vi "Construct Advanced Text Log Sink.vi"(7 "LogLevel":T3, 8 "StringFormat":refnum<class "IStringFormat.lvclass">, 9 "Log Filter":refnum<class "ILogFilter.lvclass">, 10 "Error Action":T1=enum."Ignore Error and Close Sink", 11 "Text File Configuration":T2={"Folder"=path "", "Name"="Event Log", "Extension"="txt", "Max Size (MB)"=1, "Timestamp Filename"=TRUE}) -> (3 "Text File Sink out":refnum<class "Text File Sink.lvclass">)   [LabVIEW 2018, in "MVA Framework.lvlib" / "Text File Sink.lvclass"]
doc: "Construct a text file sink. Text file configuration parameters are defined below.\n-Folder - the folder path where log files will be generated. If an empty path is supplied, a default folder path at public application data will be used.\n-Name - Name to give the log file. If no name is provided, a default file name cooresponding to the application directory name will be used.\n-Extension - file extension to be used for the log file. Note a period is not required here."
uses:
  Text File Sink.lvclass
  Composed Log/Log Sink/Log Sink.lvclass
  <vilib>/Utility/sysdir.llb/System Directory Type.ctl
  String Log Sink/String Log Sink.lvclass
  Composed Log/Types/Log Level.ctl
  Composed Log/Composed Log.lvlib
  Configuration.ctl
  Composed Log/Log Sink/Sink Error Actions ENUM.ctl
  Composed Log/ILogFilter/ILogFilter.lvclass
  IStringFormat/IStringFormat.lvclass
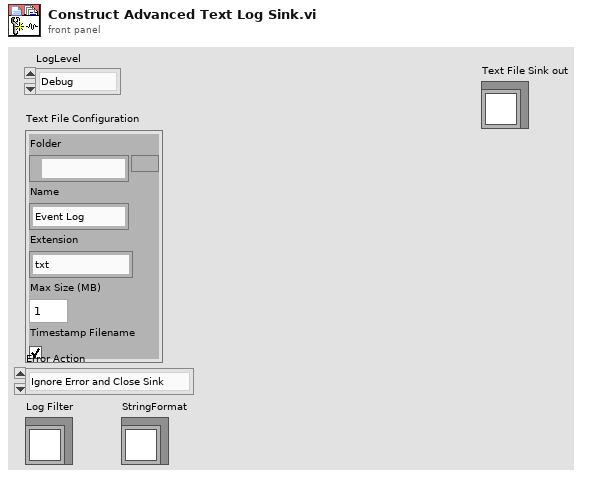
[diagram p1: front panel]
types:
  T1 = typedef "MVA Framework.lvlib/Composed Log.lvlib/Log Sink.lvclass/Sink Error Actions ENUM.ctl" = enum16{"Ignore Error and Continue", "Ignore Error and Close Sink", "Report Error and Close Sink"}
  T2 = typedef "MVA Framework.lvlib/Text File Sink.lvclass/Configuration.ctl" = cluster{"Folder":path, "Name":string, "Extension":string, "Max Size (MB)":i64, "Timestamp Filename":bool}
  T3 = typedef "MVA Framework.lvlib/Composed Log.lvlib/Log Level.ctl" = enum16{"Debug", "Info", "Warning", "Error", "Critical"}
  T4 = typedef "System Directory Type.ctl" = i32
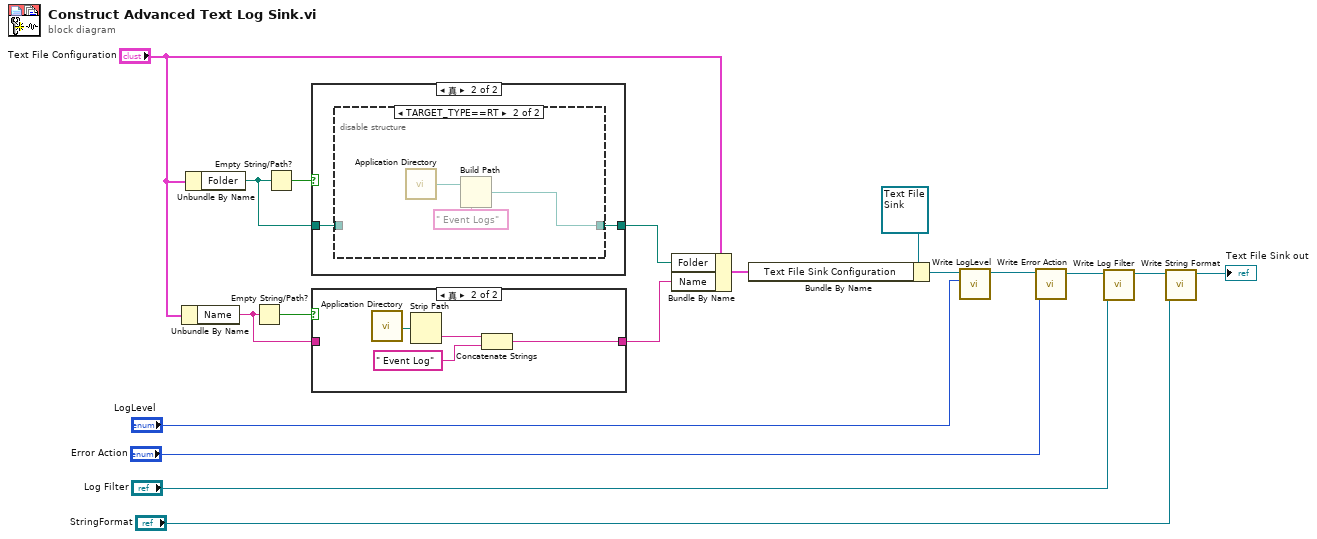
[diagram p0: block diagram]
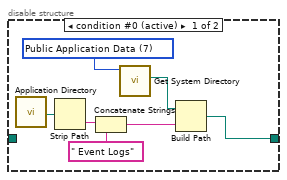
[diagram p4: hidden frame]
diagram:
  n1 = Unbundle By Name("Text File Configuration") -> ("Name"=w9:string)
  n2 = Unbundle By Name("Text File Configuration") -> ("Folder"=w11:path)
  n3 = Empty String/Path?(string/path=w9) -> (empty?=w14:bool)
  n4 = Empty String/Path?(string/path=w11) -> (empty?=w16:bool)
  n5 = case shown="真" w16 {
    tunnel: w11 -> [w19 w20]
    tunnel: [w19 w21] -> w15
    frame False {
    }
    frame True {
      n6 = disable-structure shown="TARGET_TYPE==RT" {
        disable-tunnel: [w22 w29] -> w21
        disable-tunnel: w20 -> [_ _]
        frame condition #0 (active) {
          w28 = T4 7 items=["User Home"=0, "User Desktop"=1, "User Documents"=2, "User Application Data"=3, "User Preferences"=4, "User Temporary"=5, "Public Documents"=6, "Public Application Data"=7, "Public Preferences"=8, "Public Cache"=13, "System Core Libraries"=9, "System Installed Libraries"=10, "Application Files"=11, "Boot Volume Root"=12] ("system directory type")
          n7 = call <vilib>:"Application Directory.vi"() -> ("Application Directory"=w27:path)
          n8 = Strip Path(path=w27) -> (name=w26:string)  [unwired: 1 out]
          n9 = Concatenate Strings(w26, " Event Logs" ("string")) -> (w24:string)
          n10 = call <vilib>:"Get System Directory.vi"("system directory type"=w28) -> ("system directory"=w23:path)  [unwired: 10 in]
          n11 = Build Path(base path=w23, name or relative path=w24) -> (appended path=w22:path)
        }
        frame condition #1 {
          n12 = call <vilib>:"Application Directory.vi"() -> ("Application Directory"=w30:path)
          n13 = Build Path(base path=w30, name or relative path=" Event Logs" ("string")) -> (appended path=w29:path)
        }
      }
    }
  }
  n14 = case shown="真" w14 {
    tunnel: w9 -> [w32 _]
    tunnel: [w32 w33] -> w13
    frame False {
    }
    frame True {
      n15 = call <vilib>:"Application Directory.vi"() -> ("Application Directory"=w36:path)
      n16 = Strip Path(path=w36) -> (name=w35:string)  [unwired: 1 out]
      n17 = Concatenate Strings(w35, " Event Log" ("string")) -> (w33:string)
    }
  }
  n18 = Bundle By Name(cluster="Text File Configuration", "Folder"=w15, "Name"=w13) -> (w8:T2)
  n19 = Bundle By Name(cluster=refnum<class "Text File Sink.lvclass"> refnum ("Text File Sink in"), "Text File Sink Configuration"=w8) -> (w12:refnum<class "Text File Sink.lvclass">)
  n20 = call "Write LogLevel.vi"("LogLevel"="LogLevel", "Log Sink in"=w12) -> ("Log Sink out"=w6:refnum<class "Text File Sink.lvclass">)  [unwired: 8 in, 1 out]
  n21 = call "Write Error Action.vi"("Error Action"="Error Action", "Log Sink in"=w6) -> ("Log Sink out"=w7:refnum<class "Text File Sink.lvclass">)  [unwired: 8 in, 1 out]
  n22 = call "Write Log Filter.vi"("Log Filter"="Log Filter", "Log Sink in"=w7) -> ("Log Sink out"=w3:refnum<class "Text File Sink.lvclass">)  [unwired: 8 in, 1 out]
  n23 = call "Write String Format.vi"("StringFormat"="StringFormat", "String Log Sink in"=w3) -> ("String Log Sink out"=→"Text File Sink out":refnum<class "Text File Sink.lvclass">)  [unwired: 8 in, 1 out]
